vi "vi self history.vi"() -> ()   [LabVIEW 2013]
panel:
  out "concatenated string":string
  out "array":string[](array[string])
  out "standard output":string
  out "VI Name":string
  out "History:Revision Number":u32
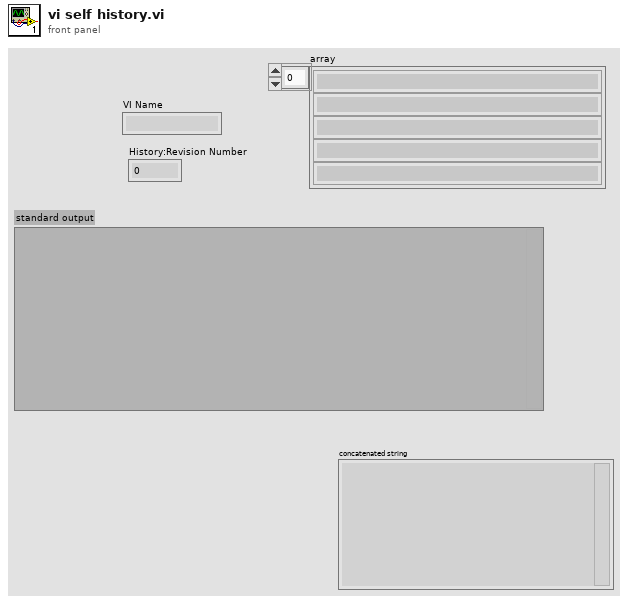
[diagram p1: front panel]
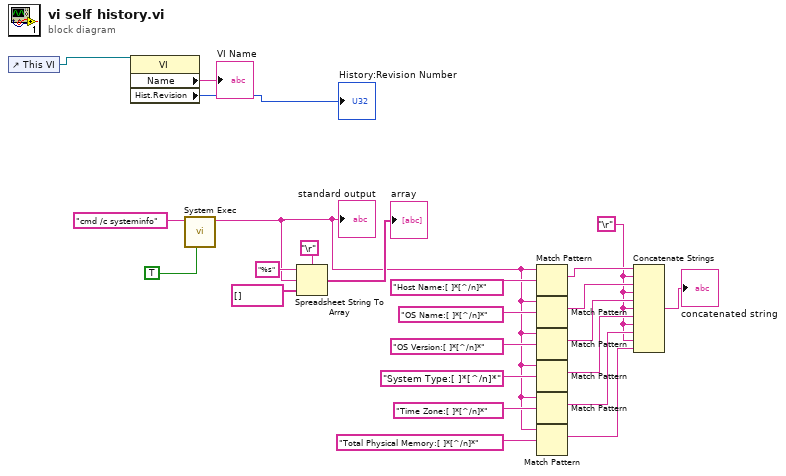
[diagram p0: block diagram]
diagram:
  w1 = "\r"
  n1 = control-ref of="This VI"() -> (w23:refnum<vi>)
  n2 = property class="VI"(reference=w23) -> ("Name"=→"VI Name":string, "Hist.Revision"=→"History:Revision Number":u32)  [unwired: 1 in, 2 out]
  n3 = call <vilib>:"System Exec.vi"("run minimized? (F)"=TRUE, "command line"="cmd /c systeminfo") -> ("standard output"=w2:string)  [unwired: 6 in, 3 out]
  "standard output" <- w2
  n4 = Spreadsheet String To Array(delimiter (Tab)="\r", format string="%s", spreadsheet string=w2, array type (2D Dbl)=string[] []) -> (array=→"array":string[])
  n5 = Match Pattern(string=w2, regular expression="Host Name:[ ]*[^/n]*") -> (match substring=w9:string)  [unwired: 1 in, 3 out]
  n6 = Match Pattern(string=w2, regular expression="OS Name:[ ]*[^/n]*") -> (match substring=w8:string)  [unwired: 1 in, 3 out]
  n7 = Match Pattern(string=w2, regular expression="OS Version:[ ]*[^/n]*") -> (match substring=w7:string)  [unwired: 1 in, 3 out]
  n8 = Match Pattern(string=w2, regular expression="System Type:[ ]*[^/n]*") -> (match substring=w6:string)  [unwired: 1 in, 3 out]
  n9 = Match Pattern(string=w2, regular expression="Time Zone:[ ]*[^/n]*") -> (match substring=w5:string)  [unwired: 1 in, 3 out]
  n10 = Match Pattern(string=w2, regular expression="Total Physical Memory:[ ]*[^/n]*") -> (match substring=w4:string)  [unwired: 1 in, 3 out]
  n11 = Concatenate Strings(w9, w1, w8, w1, w7, w1, w6, w1, w5, w1, w4) -> (→"concatenated string":string)
